vi "SubVI - no inline.vi"(1 "Array in":dbl[](array[numeric])) -> (0 "Array out":dbl[](array[numeric]))   [LabVIEW 2025]
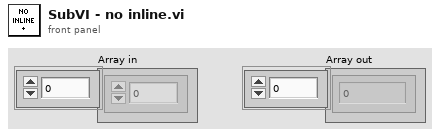
[diagram p1: front panel]
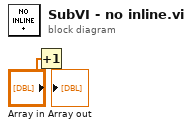
[diagram p0: block diagram]
diagram:
  n1 = Increment(x="Array in") -> (x+1=→"Array out":dbl[])
